vi "is_done.vi"(8 "error in (no error)":errorcluster, 11 "DAQmx_pulse_out in":refnum<class "DAQmx_DO.lvclass">) -> (0 "error out":errorcluster, 2 "task done?":bool, 3 "DAQmx_pulse_out out":refnum<class "DAQmx_DO.lvclass">)   [LabVIEW 2013, in "DAQmx_DO.lvclass"]
uses:
  DAQmx_DO.lvclass
  DAQmx_DO.lvclass/DAQmx_DO.ctl
  Globals.vi
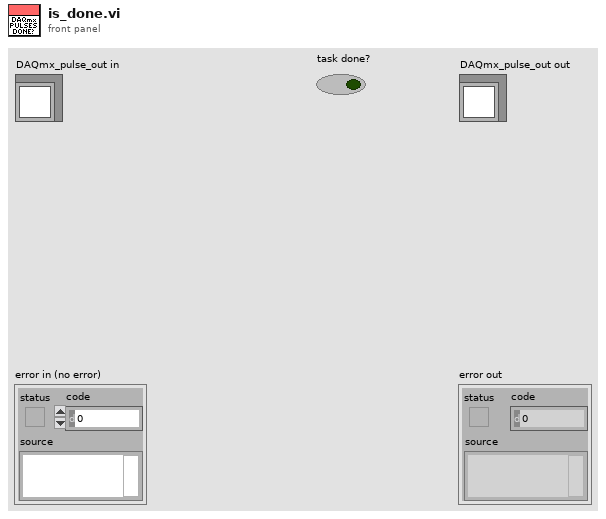
[diagram p1: front panel]
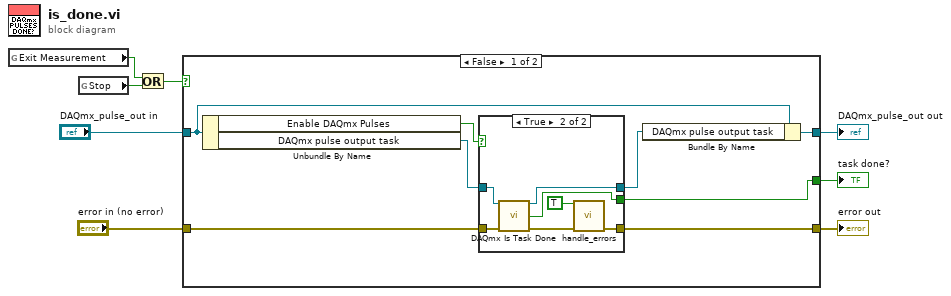
[diagram p0: block diagram]
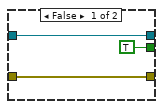
[diagram p2: hidden frame]
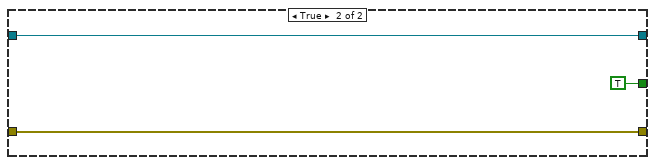
[diagram p3: hidden frame]
diagram:
  n1 = global read "Globals.vi" "Exit Measurement"() -> (w4:bool)
  n2 = global read "Globals.vi" "Stop"() -> (w3:bool)
  n3 = Or(x=w4, y=w3) -> (x .or. y?=w2:bool)
  n4 = case shown="False" w2 {
    tunnel: [w15 w28] -> w8
    tunnel: [w12 w29] -> w6
    tunnel: "DAQmx_pulse_out in" -> [w13 w29]
    tunnel: "error in (no error)" -> [w10 w28]
    tunnel: [w9 TRUE ("Exit Measurement")] -> w1
    frame False {
      n5 = Unbundle By Name(w13) -> ("Enable DAQmx Pulses"=w16:bool, "DAQmx pulse output task"=w14:refnum<k21>)
      n6 = case shown="True" w16 {
        tunnel: w10 -> [w19 w26]
        tunnel: [w19 w21] -> w15
        tunnel: w14 -> [w18 w25]
        tunnel: [w18 w24] -> w11
        tunnel: [TRUE ("task done?") w23] -> w9
        frame False {
        }
        frame True {
          n7 = call <vilib>:"DAQmx Is Task Done.vi"("task/channels in"=w25, "error in"=w26) -> ("task out"=w24:refnum<k21>, "task done?"=w23:bool, "error out"=w22:errorcluster)  [unwired: 11 in]
          n8 = call "handle_errors.vi"("Exit Operation"=TRUE ("Exit Measurement"), "error in (no error)"=w22) -> ("error out"=w21:errorcluster)  [unwired: 13 in]
        }
      }
      n9 = Bundle By Name(cluster=w13, "DAQmx pulse output task"=w11) -> (w12:refnum<class "DAQmx_DO.lvclass">)
    }
    frame True {
    }
  }
  "error out" <- w8
  "DAQmx_pulse_out out" <- w6
  "task done?" <- w1
